vi "UHR-Fleezers Control (host) - 12.2.vi"() -> ()   [LabVIEW 2012] (continued)
            n266 = while {
              tunnel: w477 -> [w482]
              tunnel: w475 -> [w481]
              tunnel: w473 -> [w480]
              tunnel: w472 -> [w479]
              tunnel: w471 -> [w478]
              stop <- w483 stop-if-true
              n267 = event shown="[0] \"Pane\": Mouse Move" {
                selector: _ -> [_ _]
                dyn-events: _ -> [_ _]
                timeout: _ -> [_ _]
                tunnel: ["Force Manip Abort" w547] -> w483
                tunnel: w482 -> [w490 _]
                tunnel: w481 -> [w488 _]
                tunnel: w480 -> [w487 _]
                tunnel: w479 -> [w486 _]
                tunnel: w478 -> [w485 _]
                event Mouse Move {
                  n268 = event-data() -> ("Time"=w491:u32, "Coords"=w492:T7)  [unwired: 3 out]
                  n269 = Less?(x=w491, y=w490) -> (x < y?=w489:bool)
                  n270 = case "Makes sure old motion events prior to mouse click aren't used" shown="False" w489 {
                    tunnel: w492 -> [w534 _]
                    tunnel: w488 -> [w535 _]
                    tunnel: w487 -> [w512 _]
                    tunnel: w486 -> [w508 _]
                    tunnel: w485 -> [w507 _]
                    frame False {
                      n271 = Subtract(x=w534, y=w535) -> (x-y=w533:T7)
                      "Coords" <- w533
                      n272 = local read "Y RF Frequency Limits (MHz)"() -> (w493:T16)
                      n273 = To Double Precision Float(number=w533) -> (double precision float=w532:cluster{"Horizontal":dbl, "Vertical":dbl})
                      n274 = Multiply(x=cluster{"Horizontal":dbl, "Vertical":dbl} {"Horizontal"=-1.0, "Vertical"=1.0}, y="Manipulation Scaling") -> (x*y=w528:cluster{"Horizontal":dbl, "Vertical":dbl})
                      n275 = local read "X RF Frequency Limits (MHz)"() -> (w494:T16)
                      n276 = Multiply(x=w532, y=w528) -> (x*y=w530:cluster{"Horizontal":dbl, "Vertical":dbl})
                      n277 = Unbundle By Name(w530) -> ("Horizontal"=w525:dbl, "Vertical"=w529:dbl)
                      n278 = Unbundle By Name(w493) -> ("Maximum"=w496:dbl, "Minimum"=w495:dbl)
                      n279 = Boolean To (0,1)(Boolean="Manip. X?") -> (0, 1=w523:i16)
                      n280 = Boolean To (0,1)(Boolean="Manip. Y?") -> (0, 1=w520:i16)
                      n281 = local read "BD 1 Frequency 2 (MHz)"() -> (w510:dbl)
                      n282 = Multiply(x=w529, y=w520) -> (x*y=w522:dbl)
                      n283 = Multiply(x=w523, y=w525) -> (x*y=w526:dbl)
                      n284 = local read "BD 2 Frequency 2 (MHz)"() -> (w509:dbl)
                      n285 = Unbundle By Name(w494) -> ("Maximum"=w498:dbl, "Minimum"=w497:dbl)
                      n286 = Add(x=w507, y=w522) -> (x+y=w500:dbl)
                      n287 = Add(x=w508, y=w526) -> (x+y=w502:dbl)
                      n288 = In Range and Coerce(upper limit=w498, x=w502, lower limit=w497) -> (coerced(x)=w501:dbl)  [unwired: 1 out]
                      n289 = In Range and Coerce(upper limit=w496, x=w500, lower limit=w495) -> (coerced(x)=w499:dbl)  [unwired: 1 out]
                      n290 = Subtract(x=w501, y=w510) -> (x-y=w519:dbl)
                      n291 = Subtract(x=w499, y=w509) -> (x-y=w518:dbl)
                      n292 = Square(x=w519) -> (x^2=w517:dbl)
                      n293 = Square(x=w518) -> (x^2=w516:dbl)
                      n294 = Add(x=w517, y=w516) -> (x+y=w515:dbl)
                      n295 = Square Root(x=w515) -> (sqrt(x)=w511:dbl)
                      n296 = In Range and Coerce(upper limit="Limit Max (MHz)", x=w511, lower limit="Limit Min (MHz)") -> (In Range?=w504:bool)  [unwired: 1 out]
                      n297 = Not(x="Limits Enable") -> (.not. x?=w503:bool)
                      n298 = Or(x=w504, y=w503) -> (x .or. y?=w505:bool)
                      n299 = case shown="True" w505 {
                        tunnel: w512 -> [_ w545]
                        tunnel: w511 -> [_ w536]
                        tunnel: w501 -> [_ w543]
                        tunnel: w510 -> [_ w542]
                        tunnel: w499 -> [_ w541]
                        tunnel: w509 -> [_ w540]
                        tunnel: w494 -> [_ w538]
                        tunnel: w493 -> [_ w537]
                        frame False {
                        }
                        frame True {
                          n300 = local read "BD 1 Frequency 3 (MHz)"() -> (w544:dbl)
                          n301 = local read "BD 2 Frequency 3 (MHz)"() -> (w539:dbl)
                          n302 = local write "Trap Delta (MHz)"(w536) -> ()
                          n303 = call "set RF board frequency - interlace.vi"("Board 2 Frequency Limits"=w537, "Board 1 Frequency Limits"=w538, "FPGA VI Reference In"=w545, "Board 2 Frequency 3 (MHz)"=w539, "Board 1 Frequency 3 (MHz)"=w544, "Board 2 Frequency 2 (MHz)"=w540, "Board 2 Frequency 1 (MHz)"=w541, "Board 1 Frequency 2 (MHz)"=w542, "Board 1 Frequency 1  (MHz)"=w543) -> ()  [unwired: 1 in, 2 out]
                          n304 = local write "BD 2 Frequency 1 (MHz)"(w541) -> ()
                          n305 = local write "BD 1 Frequency 1 (MHz)"(w543) -> ()
                        }
                      }
                    }
                    frame True {
                    }
                  }
                }
                event Mouse Up {
                  n306 = event-data() -> ("Button"=w546:u16)  [unwired: 8 out]
                  n307 = case shown="3" w546 {
                    tunnel: [FALSE TRUE] -> w547
                    frame 0, Default {
                    }
                    frame 3 {
                      n308 = local read "Trap Delta (MHz)"() -> (w549:dbl)
                      n309 = property on="Initial delta (MHz)" class="DigNum (strict)"("Val(Sgnl)"=w549) -> ()  [unwired: 2 in, 2 out]
                      n310 = local write "Manipulating Trap"(FALSE ("Manipulating Trap")) -> ()
                    }
                  }
                }
              }
            }
          }
        }
      }
      event Mouse Move {
        n311 = event-data() -> ()  [unwired: 6 out]
      }
    }
    n312 = local read "Stop All"() -> (w365:bool)
    n313 = node-c288() -> ()  [unwired: 2 out]
  }
  n314 = node-c288() -> (w2:T21)  [unwired: 4 out]
  n315 = timed-loop "Run Scripts, including: stage motion" {
    tunnel: w129 -> [w558]
    tunnel: w128 -> [w559]
    tunnel: [w559] -> w127
    tunnel: [w558] -> w126
    timing: w124 -> [_]
    timing-out: [_] -> w123
    tunnel: w109 -> [w557]
    tunnel: w110 -> [w556]
    tunnel: w56 -> [w553]
    tunnel: w55 -> [w552]
    tunnel: w54 -> [w554]
    tunnel: w53 -> [w555]
    stop <- w560 stop-if-true
    n316 = node-c288() -> ()  [unwired: 1 in, 1 out]
    n317 = event shown="[1] \"Move to Position\": Value Change" {
      selector: _ -> [_ _ _ _ _ _ _ _ _ _ _ _ _ _ _ _ _ _ _]
      dyn-events: _ -> [_ _ _ _ _ _ _ _ _ _ _ _ _ _ _ _ _ _ _]
      timeout: _ -> [_ _ _ _ _ _ _ _ _ _ _ _ _ _ _ _ _ _ _]
      tunnel: ["Set Position" "Move to Position" _ _ "Read Harvard" _ _ _ _ _ _ "Got ADig bead" "Force FB Data\nScript" _ "Got DNA bead" "Take Stepping Data" _ "Take Detection Laser\nImage" _] -> _
      tunnel: [_ _ _ _ _ _ _ _ _ _ _ _ _ _ _ _ _ _ w1177] -> w560
      tunnel: w558 -> [w578 w586 w599 w629 _ w674 w714 w795 w824 w956 w982 _ w1018 _ _ _ _ _ _]
      tunnel: w559 -> [w579 w587 w600 w630 _ w675 w715 w796 w825 w957 w983 _ w1019 _ _ _ _ _ _]
      tunnel: w557 -> [_ _ _ _ w659 _ _ _ _ _ _ _ _ _ _ _ _ _ _]
      tunnel: w556 -> [_ _ _ _ w658 _ _ _ _ _ _ _ _ _ _ _ _ _ _]
      tunnel: w555 -> [_ _ _ _ _ _ _ _ _ _ _ _ _ _ _ _ _ _ _]
      tunnel: w554 -> [_ _ _ _ _ _ _ _ _ _ _ _ _ _ _ _ _ _ _]
      tunnel: w553 -> [_ _ _ _ _ _ _ _ _ _ _ _ _ _ _ _ _ _ _]
      tunnel: w552 -> [_ _ _ _ _ _ _ _ _ _ _ _ _ _ _ _ _ _ _]
      event "Set Position", "Set Position 2", "Set Position 3", "Set Position 4", "Set Position 5", "Set Position 1": Value Change {
        n318 = event-data() -> ()  [unwired: 1 in, 5 out]
        n319 = Build Array("Set Position 1", "Set Position 2", "Set Position 3", "Set Position 4", "Set Position 5") -> (w577:bool[])
        n320 = Boolean Array To Number(Boolean array=w577) -> (number=w576:u32)
        n321 = Logarithm Base 2(1:w576) -> (0:w568:dbl)
        n322 = call "Read Stage Position.vi"("error in"=w578, "VISA resource name in"=w579) -> ("Current Position"=w583:cluster{dbl, dbl, dbl}, "error out"=w582:errorcluster)  [unwired: 2 out]
        n323 = Decrement(x="Position") -> (x-1=w566:dbl)
        n324 = Greater Or Equal?(x=w568, y=0.0) -> (x >= y?=w569:bool)
        n325 = Cluster To Array(cluster=w583) -> (array=w580:dbl[])
        n326 = local write "Stage Control Serial Error"(w582) -> ()
        n327 = Select(t=w568, s=w569, f=w566) -> (s? t:f=w565:dbl)
        n328 = Increment(x=w565) -> (x+1=w564:dbl)
        n329 = Build Array (concatenate)(w564, w580) -> (w563:dbl[])
        n330 = Replace Array Subset(array="Saved Stage Positions", new element=w563, index (row)=w565) -> (w581:dbl[][])  [unwired: 1 in]
        n331 = local write "Saved Stage Positions"(w581) -> ()
      }
      event "Move to Position": Value Change {
        n332 = event-data() -> ()  [unwired: 1 in, 5 out]
        n333 = flat-sequence {
          tunnel: w587 -> [w591]
          tunnel: w586 -> [w590]
          frame #0 {
            n334 = local read "Saved Stage Positions"() -> (w593:dbl[][])
            n335 = local read "Position"() -> (w592:dbl)
            n336 = local write "Stage Moving"(TRUE ("Stage Moving")) -> ()
            n337 = call "move to saved stage position.vi"("error in"=w590, "Stage VISA resource name in"=w591, "Position"=w592, "Saved Stage Positions"=w593) -> ("error out"=w589:errorcluster)  [unwired: 1 out]
            n338 = local write "Stage Control Serial Error"(w589) -> ()
          }
          frame #1 {
            n339 = call <vilib>:"Beep.vi"() -> ()  [unwired: 3 in, 9 out]
            n340 = local write "Stage Moving"(FALSE ("Stage Moving")) -> ()
          }
        }
      }
      event "Move Cap. 1 (DNA Bottom)": Value Change {
        n341 = event-data() -> ()  [unwired: 1 in, 5 out]
        n342 = local write "Move Cap. 1 (DNA Bottom)"(FALSE ("Move Cap. 1 (DNA Right)")) -> ()
        n343 = flat-sequence {
          tunnel: w599 -> [w602]
          tunnel: w600 -> [w603]
          tunnel: [w603] -> w597
          tunnel: [w602] -> w596
          tunnel: w597 -> [w605]
          tunnel: w596 -> [w604]
          frame #0 {
            n344 = property on="Sample Channel\nFlow" class="Bool (strict)"("Val(Sgnl)"="Cap 1 Samp Flow ON") -> ()  [unwired: 2 in, 2 out]
          }
          frame #1 {
            n345 = local read "Saved Stage Positions"() -> (w615:dbl[][])
            n346 = local write "Stage Moving"(TRUE ("Stage Moving")) -> ()
            n347 = Array Subset(array=w615, index (row)=0 ("index"), length (row)=1 ("length"), index (col)=1 ("index"), length (col)=3 ("length")) -> (w612:dbl[][])
            n348 = Reshape Array(w612, 3 ("dimension size")) -> (w610:dbl[])
            n349 = Array To Cluster(array=w610) -> (cluster=w609:cluster{"[0]":dbl, "[1]":dbl, "[2]":dbl})
            n350 = call "Set Stage Position.vi"("Position"=w609, "error in"=w604, "VISA resource name in"=w605) -> ("error out"=w608:errorcluster)  [unwired: 2 out]
            n351 = local write "Stage Control Serial Error"(w608) -> ()
          }
          frame #2 {
            n352 = local write "Stage Moving"(FALSE ("Stage Moving")) -> ()
            n353 = case shown="True" "Cap 1 Flow ON" {
              frame False {
              }
              frame True {
                n354 = property on="Inject Pump 1" class="Bool (strict)"("Val(Sgnl)"=TRUE ("Value (Signaling)")) -> ()  [unwired: 2 in, 2 out]
              }
            }
            n355 = call <vilib>:"Beep.vi"() -> ()  [unwired: 3 in, 9 out]
          }
          frame #3 {
            n356 = property on="Sample Channel\nFlow" class="Bool (strict)"("Val(Sgnl)"=FALSE ("Value (Signaling)")) -> ()  [unwired: 2 in, 2 out]
            n357 = local read "Cap. 2 BD T1?\n(ADig T1, DNA T2)"() -> (w622:bool)
            n358 = case shown="True" w622 {
              tunnel: "Cap 1 T ON" -> [w624 w625]
              frame False {
                n359 = property on="Trap 1 (ON/OFF)" class="Bool (strict)"("Val(Sgnl)"=w624) -> ()  [unwired: 2 in, 2 out]
              }
              frame True {
                n360 = property on="Trap 2 (ON/OFF)" class="Bool (strict)"("Val(Sgnl)"=w625) -> ()  [unwired: 2 in, 2 out]
              }
            }
            n361 = property on="Got DNA bead" class="Bool"("Key Focus"=TRUE) -> ()  [unwired: 2 in, 2 out]
          }
        }
      }
      event "Move Cap. 2 (ADig Top)": Value Change {
        n362 = event-data() -> ()  [unwired: 1 in, 5 out]
        n363 = local write "Move Cap. 2 (ADig Top)"(FALSE ("Move Cap. 2 (ADig Left)")) -> ()
        n364 = flat-sequence {
          tunnel: w629 -> [w632]
          tunnel: w630 -> [w633]
          tunnel: [w633] -> w627
          tunnel: [w632] -> w626
          tunnel: w627 -> [w636]
          tunnel: w626 -> [w635]
          frame #0 {
            n365 = property on="Sample Channel\nFlow" class="Bool (strict)"("Val(Sgnl)"="Cap 2 Samp Flow ON") -> ()  [unwired: 2 in, 2 out]
          }
          frame #1 {
            w634 = FALSE ("Value (Signaling)")
            n366 = local read "Saved Stage Positions"() -> (w646:dbl[][])
            n367 = local write "Stage Moving"(TRUE ("Stage Moving")) -> ()
            n368 = Array Subset(array=w646, index (row)=1 ("index"), length (row)=1 ("length"), index (col)=1 ("index"), length (col)=3 ("length")) -> (w643:dbl[][])
            n369 = Reshape Array(w643, 3 ("dimension size")) -> (w641:dbl[])
            n370 = property on="Trap 1 (ON/OFF)" class="Bool (strict)"("Val(Sgnl)"=w634) -> ()  [unwired: 2 in, 2 out]
            n371 = property on="Trap 1 (ON/OFF)" class="Bool (strict)"("Val(Sgnl)"=w634) -> ()  [unwired: 2 in, 2 out]
            n372 = Array To Cluster(array=w641) -> (cluster=w640:cluster{"[0]":dbl, "[1]":dbl, "[2]":dbl})
            n373 = call "Set Stage Position.vi"("Position"=w640, "error in"=w635, "VISA resource name in"=w636) -> ("error out"=w639:errorcluster)  [unwired: 2 out]
            n374 = local write "Stage Control Serial Error"(w639) -> ()
          }
          frame #2 {
            n375 = local write "Stage Moving"(FALSE ("Stage Moving")) -> ()
            n376 = call <vilib>:"Beep.vi"() -> ()  [unwired: 3 in, 9 out]
            n377 = case shown="True" "Cap 2 Flow ON" {
              frame False {
              }
              frame True {
                n378 = property on="Inject Pump 3" class="Bool (strict)"("Val(Sgnl)"=TRUE ("Value (Signaling)")) -> ()  [unwired: 2 in, 2 out]
              }
            }
          }
          frame #3 {
            n379 = property on="Sample Channel\nFlow" class="Bool (strict)"("Val(Sgnl)"=FALSE ("Value (Signaling)")) -> ()  [unwired: 2 in, 2 out]
            n380 = case shown="False" "Cap. 2 BD T1?\n(ADig T1, DNA T2)" {
              tunnel: "Cap 2 T ON" -> [w655 w656]
              frame False {
                n381 = property on="Trap 2 (ON/OFF)" class="Bool (strict)"("Val(Sgnl)"=w655) -> ()  [unwired: 2 in, 2 out]
              }
              frame True {
                n382 = property on="Trap 1 (ON/OFF)" class="Bool (strict)"("Val(Sgnl)"=w656) -> ()  [unwired: 2 in, 2 out]
              }
            }
            n383 = property on="Got ADig bead" class="Bool"("Key Focus"=TRUE) -> ()  [unwired: 2 in, 2 out]
          }
        }
      }
      event "Read Harvard": Value Change {
        n384 = event-data() -> ()  [unwired: 1 in, 5 out]
        n385 = Concatenate Strings("write buffer", "\r") -> (w661:string)
        n386 = VISA Write(VISA resource name=w659, write buffer=w661, error in (no error)=w658) -> (VISA resource name out=w670:refnum<visa-resource-name>, error out=w669:errorcluster)  [unwired: 1 out]
        n387 = stacked-sequence {
          tunnel: [w673] -> w668
          tunnel: w670 -> [w673]
          tunnel: w669 -> [w672]
          tunnel: [w672] -> w663
          frame #0 {
            n388 = Wait (ms)(milliseconds to wait=50) -> ()  [unwired: 1 out]
          }
        }
        n389 = property class="Instr"(reference=w668, error in=w663) -> (reference out=w667:refnum<visa-resource-name>, error out=w665:errorcluster, "Serial Settings:Number of Bytes at Serial Port"=w666:u32)
        "Serial Settings:Number of Bytes at Serial Port" <- w666
        n390 = VISA Read(VISA resource name=w667, byte count=w666, error in (no error)=w665) -> (read buffer=w664:string)  [unwired: 3 out]
        "read buffer" <- w664
        n391 = Fract/Exp String To Number(string=w664) -> ()  [unwired: 5 out]
      }
      event "+z", "-z": Value Change {
        n392 = event-data() -> ()  [unwired: 1 in, 5 out]
        n393 = flat-sequence {
          tunnel: w674 -> [w696]
          tunnel: w675 -> [w676]
          frame #0 {
            n394 = call "Read Stage Position.vi"("error in"=w696, "VISA resource name in"=w676) -> ("Current Position"=w681:cluster{dbl, dbl, dbl}, "error out"=w694:errorcluster, "VISA resource name out"=w695:refnum<visa-resource-name>)  [unwired: 1 out]
            n395 = local read "Saved Stage Positions"() -> (w705:dbl[][])
            n396 = Divide(x="z nudge increment (um)", y=1000.0) -> (x/y=w693:dbl)
            n397 = Boolean To (0,1)(Boolean="+z") -> (0, 1=w685:i16)
            n398 = Boolean To (0,1)(Boolean="-z") -> (0, 1=w686:i16)
            n399 = Array Subset(array=w705, index (row)=1 ("index"), length (row)=1 ("length"), index (col)=1 ("index"), length (col)=3 ("length")) -> (w702:dbl[][])
            n400 = Multiply(x=w685, y=w693) -> (x*y=w689:dbl)
            n401 = Multiply(x=w686, y=w693) -> (x*y=w687:dbl)
            n402 = Unbundle(w681) -> (w679:dbl, w678:dbl, w682:dbl)
            n403 = Negate(x=w687) -> (-x=w688:dbl)
            n404 = Reshape Array(w702, 3 ("dimension size")) -> (w700:dbl[])
            n405 = Add(x=w689, y=w688) -> (x+y=w690:dbl)
            n406 = Array To Cluster(array=w700) -> ()  [unwired: 1 out]
            n407 = Add(x=w690, y=w682) -> (x+y=w680:dbl)
            n408 = Bundle(cluster=w681, w679, w678, w680) -> (w677:cluster{dbl, dbl, dbl})
            n409 = call "Set Stage Position.vi"("Position"=w677, "error in"=w694, "VISA resource name in"=w695) -> ("error out"=w699:errorcluster)  [unwired: 2 out]
            n410 = local write "Stage Moving"(TRUE ("Stage Moving")) -> ()
            n411 = local write "Stage Control Serial Error"(w699) -> ()
          }
          frame #1 {
            n412 = local write "Stage Moving"(FALSE ("Stage Moving")) -> ()
            n413 = call <vilib>:"Beep.vi"() -> ()  [unwired: 3 in, 9 out]
          }
        }
      }
      event "Cal/Data Acq. Spot": Value Change {
        n414 = event-data() -> ()  [unwired: 1 in, 5 out]
        n415 = flat-sequence {
          tunnel: w714 -> [w718]
          tunnel: w715 -> [w719]
          tunnel: [w719] -> w711
          tunnel: [w718] -> w710
          tunnel: w711 -> [w724]
          tunnel: w710 -> [w723]
          tunnel: ["Cal @ (MHz)"] -> w708
          tunnel: [w728] -> w712
          tunnel: w708 -> [w728]
          tunnel: w712 -> [w737]
          tunnel: ["W/ Offset 1"] -> w709
          tunnel: w712 -> [w758]
          tunnel: w709 -> [w756]
          frame #0 {
            n416 = property on="Sample Channel\nFlow" class="Bool (strict)"("Val(Sgnl)"="Daq spot flow on") -> ()  [unwired: 2 in, 2 out]
            n417 = Wait (ms)(milliseconds to wait=u32 250) -> ()  [unwired: 1 out]
          }
          frame #1 {
            n418 = local read "Saved Stage Positions"() -> (w721:dbl[][])
            n419 = property on="Trap Delta (MHz)" class="DigNum (strict)"("Val(Sgnl)"="Cal @ (MHz)") -> ()  [unwired: 2 in, 2 out]
            n420 = local write "Stage Moving"(TRUE ("Stage Moving")) -> ()
            n421 = call "move to saved stage position.vi"("error in"=w723, "Stage VISA resource name in"=w724, "Position"="Cal Stage Position", "Saved Stage Positions"=w721) -> ("error out"=w722:errorcluster)  [unwired: 1 out]
            n422 = local write "Stage Control Serial Error"(w722) -> ()
          }
          frame #2 {
            n423 = local write "Stage Moving"(FALSE ("Stage Moving")) -> ()
            n424 = property on="Sample Channel\nFlow" class="Bool (strict)"("Val(Sgnl)"="Flow ON during cal?") -> ()  [unwired: 2 in, 2 out]
            n425 = call <vilib>:"Beep.vi"() -> ()  [unwired: 3 in, 9 out]
          }
          frame #3 {
            n426 = Wait (ms)(milliseconds to wait=u32 1000) -> ()  [unwired: 1 out]
          }
          frame #4 {
            n427 = property on="Save Calibration" class="Bool (strict)"("Val(Sgnl)"=TRUE ("Value (Signaling)")) -> ()  [unwired: 2 in, 2 out]
          }
          frame #5 {
            n428 = Wait (ms)(milliseconds to wait=u32 2000) -> ()  [unwired: 1 out]
          }
          frame #6 {
            # "Check to see if \nsaving done"
            n429 = while {
              stop <- w733 stop-if-true
              n430 = local read "Saving..."() -> (w734:bool)
              n431 = Wait (ms)(milliseconds to wait=u32 100) -> ()  [unwired: 1 out]
              n432 = Not(x=w734) -> (.not. x?=w733:bool)
            }
          }
          frame #7 {
            n433 = case shown="True" "W/ Offset 1" {
              tunnel: w737 -> [_ w738]
              frame False {
              }
              frame True {
                n434 = stacked-sequence {
                  tunnel: w738 -> [_ _ _ _ _ _ _ w755]
                  frame #0 {
                    n435 = property on="Trap Delta (MHz)" class="DigNum (strict)"("Val(Sgnl)"="Offset 1 Start (MHz)") -> ()  [unwired: 2 in, 2 out]
                    n436 = Replace Array Subset(array=u32[] [0] ("Index Values"), new element="Offset 1 Set", index=0) -> (w739:u32[])
                    n437 = property on="Saved AOD Raster Scan Parameter Sets" class="Arr (strict)"("Index Values"=w739) -> ()  [unwired: 2 in, 2 out]
                  }
                  frame #1 {
                    n438 = Wait (ms)(milliseconds to wait=u32 200) -> ()  [unwired: 1 out]
                  }
                  frame #2 {
                    n439 = property on="Load parameters" class="Bool (strict)"("Val(Sgnl)"=TRUE ("Value (Signaling)")) -> ()  [unwired: 2 in, 2 out]
                  }
                  frame #3 {
                    n440 = Wait (ms)(milliseconds to wait=u32 200) -> ()  [unwired: 1 out]
                  }
                  frame #4 {
                    n441 = property on="Trap Raster Scan" class="Bool (strict)"("Val(Sgnl)"=TRUE ("Value (Signaling)")) -> ()  [unwired: 2 in, 2 out]
                  }
                  frame #5 {
                    n442 = Wait (ms)(milliseconds to wait=u32 2000) -> ()  [unwired: 1 out]
                  }
                  frame #6 {
                    n443 = while {
                      stop <- w752 stop-if-true
                      n444 = local read "Raster Scanning..."() -> (w754:bool)
                      n445 = local read "Saving..."() -> (w750:bool)
                      n446 = Wait (ms)(milliseconds to wait=u32 100) -> ()  [unwired: 1 out]
                      n447 = Not(x=w750) -> (.not. x?=w749:bool)
                      n448 = Not(x=w754) -> (.not. x?=w751:bool)
                      n449 = And(x=w751, y=w749) -> (x .and. y?=w752:bool)
                    }
                  }
                  frame #7 {
                    n450 = property on="Trap Delta (MHz)" class="DigNum (strict)"("Val(Sgnl)"=w755) -> ()  [unwired: 2 in, 2 out]
                  }
                }
              }
            }
          }
          frame #8 {
            n451 = local read "Save ave N"() -> (w757:dbl)
            n452 = case shown="False" "W/ Offset 2" {
              tunnel: w758 -> [_ w765]
              tunnel: w757 -> [_ w764]
              tunnel: w756 -> [w760 _]
              frame False {
                n453 = case shown="False" w760 {
                  frame False {
                    n454 = Multiply(x="Cal read wait (s)", y=u32 1000 ("milliseconds to wait")) -> (x*y=w762:u32)
                    n455 = Wait (ms)(milliseconds to wait=w762) -> ()  [unwired: 1 out]
                  }
                  frame True {
                  }
                }
              }
              frame True {
                n456 = stacked-sequence {
                  tunnel: w765 -> [_ _ _ _ _ _ _ _ _ w786 _ _]
                  tunnel: w764 -> [_ _ _ _ _ _ _ _ _ w784 _ _]
                  frame #0 {
                    n457 = property on="Save ave N" class="DigNum (strict)"("Val(Sgnl)"=1.0 ("Value (Signaling)")) -> ()  [unwired: 2 in, 2 out]
                  }
                  frame #1 {
                    n458 = Wait (ms)(milliseconds to wait=u32 500) -> ()  [unwired: 1 out]
                  }
                  frame #2 {
                    n459 = property on="Trap Delta (MHz)" class="DigNum (strict)"("Val(Sgnl)"="Offset 2 Start (MHz)") -> ()  [unwired: 2 in, 2 out]
                    n460 = Replace Array Subset(array=u32[] [0] ("Index Values"), new element="Offset 2 Set", index=0) -> (w770:u32[])
                    n461 = property on="Saved AOD Raster Scan Parameter Sets" class="Arr (strict)"("Index Values"=w770) -> ()  [unwired: 2 in, 2 out]
                  }
                  frame #3 {
                    n462 = Wait (ms)(milliseconds to wait=u32 500) -> ()  [unwired: 1 out]
                  }
                  frame #4 {
                    n463 = property on="Load parameters" class="Bool (strict)"("Val(Sgnl)"=TRUE ("Value (Signaling)")) -> ()  [unwired: 2 in, 2 out]
                  }
                  frame #5 {
                    n464 = Wait (ms)(milliseconds to wait=u32 500) -> ()  [unwired: 1 out]
                  }
                  frame #6 {
                    n465 = property on="Trap Raster Scan" class="Bool (strict)"("Val(Sgnl)"=TRUE ("Value (Signaling)")) -> ()  [unwired: 2 in, 2 out]
                  }
                  frame #7 {
                    n466 = Wait (ms)(milliseconds to wait=u32 2000) -> ()  [unwired: 1 out]
                  }
                  frame #8 {
                    n467 = while {
                      stop <- w779 stop-if-true
                      n468 = local read "Raster Scanning..."() -> (w782:bool)
                      n469 = local read "Saving..."() -> (w780:bool)
                      n470 = Wait (ms)(milliseconds to wait=u32 100) -> ()  [unwired: 1 out]
                      n471 = Not(x=w780) -> (.not. x?=w778:bool)
                      n472 = Not(x=w782) -> (.not. x?=w781:bool)
                      n473 = And(x=w781, y=w778) -> (x .and. y?=w779:bool)
                    }
                  }
                  frame #9 {
                    n474 = property on="Trap Delta (MHz)" class="DigNum (strict)"("Val(Sgnl)"=w786) -> ()  [unwired: 2 in, 2 out]
                    n475 = property on="Saved AOD Raster Scan Parameter Sets" class="Arr (strict)"("Index Values"=u32[] [0]) -> ()  [unwired: 2 in, 2 out]
                    n476 = property on="Save ave N" class="DigNum (strict)"("Val(Sgnl)"=w784) -> ()  [unwired: 2 in, 2 out]
                  }
                  frame #10 {
                    n477 = Wait (ms)(milliseconds to wait=u32 500) -> ()  [unwired: 1 out]
                  }
                  frame #11 {
                    n478 = property on="Load parameters" class="Bool (strict)"("Val(Sgnl)"=TRUE ("Value (Signaling)")) -> ()  [unwired: 2 in, 2 out]
                  }
                }
              }
            }
          }
          frame #9 {
            n479 = property on="Read Cal" class="Bool (strict)"("Val(Sgnl)"=TRUE ("Value (Signaling)")) -> ()  [unwired: 2 in, 2 out]
          }
          frame #10 {
            n480 = Wait (ms)(milliseconds to wait=u32 1000) -> ()  [unwired: 1 out]
          }
          frame #11 {
            n481 = property on="Fish for Tether" class="Bool (strict)"("Val(Sgnl)"=TRUE ("Value (Signaling)")) -> ()  [unwired: 2 in, 2 out]
          }
        }
        n482 = local write "Cal/Data Acq. Spot"(FALSE ("Cal/Data Acq. Spot")) -> ()
      }
      event "Dump Beads": Value Change {
        n483 = event-data() -> ()  [unwired: 1 in, 5 out]
        n484 = flat-sequence {
          tunnel: ["Dump spot flow on?"] -> w792
          tunnel: [w803] -> w793
          tunnel: w792 -> [w803]
          tunnel: w796 -> [w808]
          tunnel: w795 -> [w807]
          tunnel: [w805] -> w794
          tunnel: w793 -> [w805]
          tunnel: w794 -> [w818]
          frame #0 {
            w797 = FALSE ("Value (Signaling)")
            n485 = local read "Saving..."() -> (w799:bool)
            n486 = local write "Dump Beads"(FALSE ("Dump Beads")) -> ()
            n487 = property on="Inject Pump 3" class="Bool (strict)"("Val(Sgnl)"=w797) -> ()  [unwired: 2 in, 2 out]
            n488 = property on="Inject Pump 1" class="Bool (strict)"("Val(Sgnl)"=w797) -> ()  [unwired: 2 in, 2 out]
            n489 = local write "Stop Saving"(w799) -> ()
          }
          frame #1 {
            w800 = FALSE ("Fl. Triggered...")
            n490 = case shown="True" "Dump spot flow on?" {
              frame False {
              }
              frame True {
                n491 = property on="Sample Channel\nFlow" class="Bool (strict)"("Val(Sgnl)"=TRUE ("Stage Moving")) -> ()  [unwired: 2 in, 2 out]
              }
            }
            n492 = local write "Fl. Triggered..."(w800) -> ()
            n493 = local write "Tether"(w800) -> ()
            n494 = property on="Green Laser ON/Interlacing" class="Bool (strict)"("Val(Sgnl)"=w800) -> ()  [unwired: 2 in, 2 out]
            n495 = property on="Trap Pos. FB ON" class="Bool (strict)"("Val(Sgnl)"=w800) -> ()  [unwired: 2 in, 2 out]
            n496 = property on="Trap Trig. Fl." class="Bool (strict)"("Val(Sgnl)"=w800) -> ()  [unwired: 2 in, 2 out]
            n497 = property on="Fl. Triggered..." class="Bool (strict)"("Val(Sgnl)"=w800) -> ()  [unwired: 2 in, 2 out]
            n498 = property on="Dip for Protein" class="Bool (strict)"("Val(Sgnl)"=w800) -> ()  [unwired: 2 in, 2 out]
            n499 = property on="Pause dwell" class="Bool (strict)"("Val(Sgnl)"=w800) -> ()  [unwired: 2 in, 2 out]
          }
          frame #2 {
            n500 = property on="Trap Pos. FB Offset Factor" class="DigNum (strict)"("Val(Sgnl)"=i64 0 ("Value (Signaling)")) -> ()  [unwired: 2 in, 2 out]
          }
          frame #3 {
            n501 = local read "Saved Stage Positions"() -> (w809:dbl[][])
            n502 = local write "Stage Moving"(TRUE ("Stage Moving")) -> ()
            n503 = Array Subset(array=w809, index (row)=3 ("index"), length (row)=1 ("length"), index (col)=1 ("index"), length (col)=3 ("length")) -> (w814:dbl[][])
            n504 = Reshape Array(w814, 3 ("dimension size")) -> (w812:dbl[])
            n505 = Array To Cluster(array=w812) -> (cluster=w811:cluster{"[0]":dbl, "[1]":dbl, "[2]":dbl})
            n506 = call "Set Stage Position.vi"("Position"=w811, "error in"=w807, "VISA resource name in"=w808) -> ()  [unwired: 3 out]
          }
          frame #4 {
            w819 = FALSE ("Value (Signaling)")
            n507 = case shown="True" w818 {
              frame False {
              }
              frame True {
                n508 = property on="Sample Channel\nFlow" class="Bool (strict)"("Val(Sgnl)"=FALSE ("Stage Moving")) -> ()  [unwired: 2 in, 2 out]
              }
            }
            n509 = property on="Trap 1 (ON/OFF)" class="Bool (strict)"("Val(Sgnl)"=w819) -> ()  [unwired: 2 in, 2 out]
            n510 = property on="Trap 2 (ON/OFF)" class="Bool (strict)"("Val(Sgnl)"=w819) -> ()  [unwired: 2 in, 2 out]
            n511 = call <vilib>:"Beep.vi"() -> ()  [unwired: 3 in, 9 out]
          }
          frame #5 {
            n512 = property on="Move Cap. 2 (ADig Top)" class="Bool (strict)"("Val(Sgnl)"=TRUE ("Value (Signaling)")) -> ()  [unwired: 2 in, 2 out]
            n513 = property on="Tab Control" class="TabCtl (strict)"("Val(Sgnl)"=T4."Status" ("Value (Signaling)")) -> ()  [unwired: 2 in, 2 out]
          }
        }
      }
      event "Dip for Protein": Value Change {
        n514 = event-data() -> ()  [unwired: 1 in, 5 out]
        n515 = case shown="True" "Dip for Protein" {
          tunnel: w825 -> [_ w827]
          tunnel: w824 -> [_ w826]
          frame False {
          }
          frame True {
            n516 = while {
              tunnel: w827 -> [w838]
              tunnel: w826 -> [w837]
              i -> [w832]
              stop <- w834 stop-if-true
              n517 = Increment(x=w832) -> (x+1=→"Dip #":i32)
              n518 = flat-sequence {
                tunnel: w837 -> [w849]
                tunnel: w838 -> [w850]
                tunnel: [w850] -> w842
                tunnel: [w849] -> w841
                tunnel: [w843] -> w828
                tunnel: [w855] -> w836
                tunnel: [w856] -> w835
                tunnel: w842 -> [w857]
                tunnel: w841 -> [w858]
                tunnel: [w853] -> w829
                tunnel: w828 -> [w853]
                tunnel: [w866] -> w840
                tunnel: w836 -> [w866]
                tunnel: [w865] -> w839
                tunnel: w835 -> [w865]
                tunnel: [w862] -> w833
                tunnel: [w861] -> w830
                tunnel: w829 -> [w861]
                tunnel: w839 -> [w886]
                tunnel: w840 -> [w887]
                tunnel: w833 -> [w888]
                tunnel: w830 -> [w885]
                tunnel: [w944] -> w834
                frame #0 {
                  n519 = local read "Trap Pos. FB ON"() -> (w843:bool)
                  n520 = Compound Arithmetic op=AND("Flow ON\nduring dip?", "FB OFF when \nflow ON", w843) -> (w844:bool)
                  n521 = case shown="True" "Move trap \nbefore dip move?" {
                    frame False {
                    }
                    frame True {
                      n522 = property on="Trap Delta (MHz)" class="DigNum (strict)"("Val(Sgnl)"="Dipping Delta (MHz)") -> ()  [unwired: 2 in, 2 out]
                    }
                  }
                  n523 = property on="Green Laser ON/Interlacing" class="Bool (strict)"("Val(Sgnl)"="Green ON\nbefore dip?") -> ()  [unwired: 2 in, 2 out]
                  n524 = property on="Sample Channel\nFlow" class="Bool (strict)"("Val(Sgnl)"="Flow ON\nduring dip?") -> ()  [unwired: 2 in, 2 out]
                  n525 = case shown="True" w844 {
                    frame False {
                    }
                    frame True {
                      n526 = property on="Trap Pos. FB ON" class="Bool (strict)"("Val(Sgnl)"=FALSE ("Value (Signaling)")) -> ()  [unwired: 2 in, 2 out]
                    }
                  }
                }
                frame #1 {
                  n527 = local read "Saved Stage Positions"() -> (w860:dbl[][])
                  n528 = local write "Cancel dwell"(FALSE ("Cancel dwell")) -> ()
                  n529 = call "move to saved stage position.vi"("error in"=w858, "Stage VISA resource name in"=w857, "Position"="Dip Stage \nPosition", "Saved Stage Positions"=w860) -> ("VISA resource name out"=w855:refnum<visa-resource-name>, "error out"=w856:errorcluster)
                }
                frame #2 {
                  n530 = node-c288() -> (w864:T21)  [unwired: 4 in]
                  n531 = timed-loop {
                    timing: w864 -> [_]
                    timing-out: [_] -> w863
                    tunnel: [w870] -> w862
                    i -> [w867]
                    stop <- w871 stop-if-true
                    n532 = node-c288() -> ()  [unwired: 1 in, 1 out]
                    n533 = Greater Or Equal?(x=w867, y="Dip Duration (s)") -> (x >= y?=w879:bool)
                    n534 = local read "Dip for Protein"() -> (w872:bool)
                    n535 = local read "Dump Beads"() -> (w869:bool)
                    n536 = local read "Cancel dwell"() -> (w878:bool)
                    n537 = local read "Pause dwell"() -> (w875:bool)
                    n538 = Not(x=w872) -> (.not. x?=w877:bool)
                    n539 = Compound Arithmetic op=OR(w878, w879, w877) -> (w876:bool)
                    n540 = Select(t=FALSE, s=w875, f=w876) -> (s? t:f=w873:bool)
                    n541 = Not(x=w869) -> (.not. x?=w868:bool)
                    n542 = node-c288() -> ()  [unwired: 1 in, 1 out]
                    n543 = And(x=w872, y=w868) -> (x .and. y?=w870:bool)
                    n544 = Or(x=w873, y=w869) -> (x .or. y?=w871:bool)
                    "Dip Time (s)" <- w867
                  }
                  n545 = node-c288(w863) -> ()  [unwired: 1 out]
                }
                frame #3 {
                  n546 = case shown="True" w888 {
                    tunnel: w887 -> [_ w893]
                    tunnel: w886 -> [_ w892]
                    tunnel: w885 -> [_ w889]
                    frame False {
                    }
                    frame True {
                      n547 = flat-sequence {
                        tunnel: w892 -> [w897]
                        tunnel: w893 -> [w898]
                        tunnel: [w898] -> w891
                        tunnel: [w897] -> w890
                        tunnel: w889 -> [w894]
                        tunnel: w891 -> [w908]
                        tunnel: w890 -> [w907]
                        tunnel: w889 -> [w916]
                        frame #0 {
                          n548 = local read "Sample Channel\nFlow"() -> (w896:bool)
                          n549 = case shown="True" w896 {
                            tunnel: "Flow ON \nduring return\nfrom dip?" -> [w899 w902]
                            tunnel: w894 -> [_ w901]
                            frame False {
                              n550 = case shown="True" w899 {
                                frame False {
                                }
                                frame True {
                                n551 = property on="Sample Channel\nFlow" class="Bool (strict)"("Val(Sgnl)"=TRUE ("Value (Signaling)")) -> ()  [unwired: 2 in, 2 out]
                                }
                              }
                            }
                            frame True {
                              n552 = case shown="False" w902 {
                                tunnel: w901 -> [w903 _]
                                frame False {
                                n553 = property on="Trap Pos. FB ON" class="Bool (strict)"("Val(Sgnl)"=w903) -> ()  [unwired: 2 in, 2 out]
                                n554 = property on="Sample Channel\nFlow" class="Bool (strict)"("Val(Sgnl)"=FALSE ("Value (Signaling)")) -> ()  [unwired: 2 in, 2 out]
                                }
                                frame True {
                                }
                              }
                            }
                          }
                        }
                        frame #1 {
                          # "For turning on green laser before stage reaches lower spot"
                          n555 = case shown="True" "Green ON\nafter start\nreturn?" {
                            frame False {
                            }
                            frame True {
                              n556 = flat-sequence {
                                frame #0 {
                                n557 = Multiply(x="Green delay after \nstart return (s)", y=1000.0) -> (x*y=w913:dbl)
                                n558 = Wait (ms)(milliseconds to wait=w913) -> ()  [unwired: 1 out]
                                }
                                frame #1 {
                                n559 = property on="Green Laser ON/Interlacing" class="Bool (strict)"("Val(Sgnl)"=TRUE ("Value (Signaling)")) -> ()  [unwired: 2 in, 2 out]
                                }
                              }
                            }
                          }
                          n560 = local read "Saved Stage Positions"() -> (w911:dbl[][])
                          n561 = local write "Cancel dwell"(FALSE ("Cancel dwell")) -> ()
                          n562 = call "move to saved stage position.vi"("error in"=w907, "Stage VISA resource name in"=w908, "Position"="Return Stage \nPosition", "Saved Stage Positions"=w911) -> ("error out"=w909:errorcluster)  [unwired: 1 out]
                          n563 = local write "Stage Control Serial Error"(w909) -> ()
                        }
                        frame #2 {
                          n564 = property on="Trap Pos. FB ON" class="Bool (strict)"("Val(Sgnl)"=w916) -> ()  [unwired: 2 in, 2 out]
                          n565 = case shown="True" "Green ON \nafter return?" {
                            frame False {
                            }
                            frame True {
                              n566 = property on="Green Laser ON/Interlacing" class="Bool (strict)"("Val(Sgnl)"=TRUE ("Value (Signaling)")) -> ()  [unwired: 2 in, 2 out]
                            }
                          }
                          n567 = case shown="True" "Move trap after return?" {
                            frame False {
                            }
                            frame True {
                              n568 = property on="Trap Delta (MHz)" class="DigNum (strict)"("Val(Sgnl)"="Dip Trap Delta 2 (MHz)") -> ()  [unwired: 2 in, 2 out]
                            }
                          }
                          n569 = case shown="True" "Save data after return?" {
                            frame False {
                            }
                            frame True {
                              n570 = property on="Start Saving" class="Bool (strict)"("Val(Sgnl)"=TRUE ("Value (Signaling)")) -> ()  [unwired: 2 in, 2 out]
                            }
                          }
                          n571 = property on="Sample Channel\nFlow" class="Bool (strict)"("Val(Sgnl)"="Flow ON\nduring daq?") -> ()  [unwired: 2 in, 2 out]
                        }
                        frame #3 {
                          n572 = node-c288() -> (w925:T21)  [unwired: 4 in]
                          n573 = timed-loop {
                            timing: w925 -> [_]
                            timing-out: [_] -> w924
                            i -> [w926]
                            stop <- w928 stop-if-true
                            n574 = node-c288() -> ()  [unwired: 1 in, 1 out]
                            n575 = local read "Dump Beads"() -> (w927:bool)
                            n576 = Greater Or Equal?(x=w926, y="Dwell Duration (s)") -> (x >= y?=w933:bool)
                            n577 = local read "Dip for Protein"() -> (w930:bool)
                            n578 = Not(x=w930) -> (.not. x?=w929:bool)
                            n579 = Compound Arithmetic op=OR(w933, "Cancel dwell", w929) -> (w932:bool)
                            n580 = node-c288() -> ()  [unwired: 1 in, 1 out]
                            n581 = Select(t=FALSE, s="Pause dwell", f=w932) -> (s? t:f=w935:bool)
                            n582 = Or(x=w935, y=w927) -> (x .or. y?=w928:bool)
                            "Dwell Time (s)" <- w926
                          }
                          n583 = node-c288(w924) -> ()  [unwired: 1 out]
                        }
                      }
                    }
                  }
                }
                frame #4 {
                  n584 = local read "Dip for Protein"() -> (w945:bool)
                  n585 = local read "Dump Beads"() -> (w942:bool)
                  n586 = local write "Cancel dwell"(FALSE ("Cancel dwell")) -> ()
                  n587 = Not(x=w945) -> (.not. x?=w946:bool)
                  n588 = Not(x="Cont. Repeat Dipping?") -> (.not. x?=w948:bool)
                  n589 = Compound Arithmetic op=OR(w946, w948, w942) -> (w944:bool)
                }
              }
            }
          }
        }
      }
      event "Profile": Value Change {
        n590 = event-data() -> ()  [unwired: 1 in, 5 out]
        n591 = flat-sequence {
          tunnel: w957 -> [w960]
          tunnel: w956 -> [w968]
          tunnel: [w962] -> w955
          tunnel: [w961] -> w954
          tunnel: [w959] -> w952
          tunnel: [w958] -> w949
          tunnel: w955 -> [w975]
          tunnel: w954 -> [w974]
          tunnel: [w972] -> w953
          tunnel: w952 -> [w973]
          tunnel: [w971] -> w951
          tunnel: [w970] -> w950
          tunnel: w949 -> [w970]
          tunnel: w953 -> [w979]
          tunnel: w951 -> [w978]
          tunnel: w950 -> [w977]
          frame #0 {
            n592 = call "Read Stage Position.vi"("error in"=w968, "VISA resource name in"=w960) -> ("Current Position"=w958:cluster{dbl, dbl, dbl}, "error out"=w961:errorcluster, "VISA resource name out"=w959:refnum<visa-resource-name>)  [unwired: 1 out]
            "Current Position" <- w958
            n593 = local write "Stage Control Serial Error"(w961) -> ()
            n594 = Unbundle(w958) -> (w965:dbl, w967:dbl, w963:dbl)
            n595 = Add(x=w967, y="Y change (mm)") -> (x+y=w964:dbl)
            n596 = Bundle(w965, w964, w963) -> (w962:cluster{dbl, dbl, dbl})  [unwired: 1 in]
          }
          frame #1 {
            # "move to new position and start saving"
            n597 = local write "Stage Moving"(TRUE ("Stage Moving")) -> ()
            n598 = local write "Start Saving"(TRUE ("Start Saving")) -> ()
            n599 = call "Set Stage Position.vi"("Position"=w975, "error in"=w974, "VISA resource name in"=w973) -> ("error out"=w971:errorcluster, "VISA resource name out"=w972:refnum<visa-resource-name>)  [unwired: 1 out]
          }
          frame #2 {
            # "go back to start"
            n600 = call "Set Stage Position.vi"("Position"=w977, "error in"=w978, "VISA resource name in"=w979) -> ()  [unwired: 3 out]
          }
          frame #3 {
            # "stop saving"
            n601 = local write "Stop Saving"(TRUE ("Stop Saving")) -> ()
            n602 = local write "Stage Moving"(FALSE ("Stage Moving")) -> ()
          }
        }
      }
      event "Move to Position 1", "Move to Position 2", "Move to Position 3", "Move to Position 4", "Move to Position 5", "Lower Ch. Cap.": Value Change {
        n603 = event-data() -> ()  [unwired: 1 in, 5 out]
        n604 = Or(x="Move to Position 5", y="Lower Ch. Cap.") -> (x .or. y?=w985:bool)
        n605 = Build Array("Move to Position 1", "Move to Position 2", "Move to Position 3", "Move to Position 4", w985) -> (w988:bool[])
        n606 = Boolean Array To Number(Boolean array=w988) -> (number=w987:u32)
        n607 = Logarithm Base 2(1:w987) -> (0:w986:dbl)
        n608 = flat-sequence {
          tunnel: w986 -> [w997]
          tunnel: w983 -> [w995]
          tunnel: w982 -> [w994]
          frame #0 {
            n609 = local read "Saved Stage Positions"() -> (w1005:dbl[][])
            n610 = Array Subset(array=w1005, index (row)=w997, length (row)=1 ("length"), index (col)=1 ("index"), length (col)=3 ("length")) -> (w1002:dbl[][])
            n611 = Reshape Array(w1002, 3 ("dimension size")) -> (w1000:dbl[])
            n612 = Array To Cluster(array=w1000) -> (cluster=w999:cluster{"[0]":dbl, "[1]":dbl, "[2]":dbl})
            n613 = call "Set Stage Position.vi"("Position"=w999, "error in"=w994, "VISA resource name in"=w995) -> ("error out"=w998:errorcluster)  [unwired: 2 out]
            n614 = local write "Stage Moving"(TRUE ("Stage Moving")) -> ()
            n615 = local write "Stage Control Serial Error"(w998) -> ()
          }
          frame #1 {
            n616 = local write "Stage Moving"(FALSE ("Stage Moving")) -> ()
            n617 = call <vilib>:"Beep.vi"() -> ()  [unwired: 3 in, 9 out]
          }
        }
      }
      event "Got ADig bead": Value Change {
        n618 = event-data() -> ()  [unwired: 1 in, 5 out]
        n619 = flat-sequence {
          frame #0 {
            n620 = local read "Cap 1 Samp Flow ON"() -> (w1009:bool)
            n621 = case shown="True" w1009 {
              frame False {
              }
              frame True {
                n622 = property on="Sample Channel\nFlow" class="Bool (strict)"("Val(Sgnl)"=TRUE ("Value (Signaling)")) -> ()  [unwired: 2 in, 2 out]
              }
            }
          }
          frame #1 {
            n623 = property on="Inject Pump 3" class="Bool (strict)"("Val(Sgnl)"=FALSE ("Value (Signaling)")) -> ()  [unwired: 2 in, 2 out]
          }
          frame #2 {
            n624 = property on="Move Cap. 1 (DNA Bottom)" class="Bool (strict)"("Val(Sgnl)"=TRUE ("Value (Signaling)")) -> ()  [unwired: 2 in, 2 out]
          }
        }
      }
      event "Force FB Data\nScript": Value Change {
        n625 = event-data() -> ()  [unwired: 1 in, 5 out]
        n626 = flat-sequence {
          tunnel: w1018 -> [w1022]
          tunnel: w1019 -> [w1023]
          tunnel: [w1023] -> w1014
          tunnel: [w1022] -> w1013
          tunnel: w1014 -> [w1026]
          tunnel: w1013 -> [w1025]
          tunnel: ["Trap Trig Fl."] -> w1015
          tunnel: [w1051] -> w1016
          tunnel: w1015 -> [w1051]
          tunnel: [w1055] -> w1017
          tunnel: w1016 -> [w1055]
          tunnel: w1017 -> [w1057]
          frame #0 {
            n627 = property on="Trap Delta (MHz)" class="DigNum (strict)"("Val(Sgnl)"="Trap Delta Before Moving") -> ()  [unwired: 2 in, 2 out]
          }
          frame #1 {
            n628 = local read "Saved Stage Positions"() -> (w1028:dbl[][])
            n629 = local write "FB Trap Pos Offset"(0.0 ("FB Trap Pos Offset")) -> ()
            n630 = property on="Trap Pos. FB Offset Factor" class="DigNum (strict)"("Val(Sgnl)"=i64 0 ("Value (Signaling)")) -> ()  [unwired: 2 in, 2 out]
            n631 = local write "Stage Moving"(TRUE ("Stage Moving")) -> ()
            n632 = call "move to saved stage position.vi"("error in"=w1025, "Stage VISA resource name in"=w1026, "Position"="Stage Position To Establish FB", "Saved Stage Positions"=w1028) -> ("error out"=w1024:errorcluster)  [unwired: 1 out]
            n633 = local write "Stage Control Serial Error"(w1024) -> ()
          }
          frame #2 {
            n634 = call <vilib>:"Beep.vi"() -> ()  [unwired: 3 in, 9 out]
            n635 = Multiply(x="Wait (s)", y=u32 1000 ("milliseconds to wait")) -> (x*y=w1035:u32)
            n636 = property on="Trap Delta (MHz)" class="DigNum (strict)"("Val(Sgnl)"="Starting \nTrap Delta (MHz)") -> ()  [unwired: 2 in, 2 out]
            n637 = local write "Stage Moving"(FALSE ("Stage Moving")) -> ()
            n638 = Wait (ms)(milliseconds to wait=w1035) -> ()  [unwired: 1 out]
            n639 = property on="Tab Control 2" class="TabCtl (strict)"("Val(Sgnl)"=T6."Feedback on Trap Position" ("Value (Signaling)")) -> ()  [unwired: 2 in, 2 out]
            n640 = property on="Tab Control" class="TabCtl (strict)"("Val(Sgnl)"=T4."Trap Control (RF)" ("Value (Signaling)")) -> ()  [unwired: 2 in, 2 out]
          }
          frame #3 {
            n641 = property on="Set Reading to\nSetpoint" class="Bool (strict)"("Val(Sgnl)"=TRUE ("Value (Signaling)")) -> ()  [unwired: 2 in, 2 out]
            n642 = Wait (ms)(milliseconds to wait=u32 500) -> ()  [unwired: 1 out]
          }
          frame #4 {
            n643 = property on="Trap Pos. FB ON" class="Bool (strict)"("Val(Sgnl)"=TRUE ("Value (Signaling)")) -> ()  [unwired: 2 in, 2 out]
            n644 = Wait (ms)(milliseconds to wait=u32 250) -> ()  [unwired: 1 out]
          }
          frame #5 {
            n645 = case shown="False" "Trap Trig Fl." {
              frame False {
                n646 = case shown="True" "Green ON after FB ON?" {
                  selector: "Green ON after FB ON?" -> [_ w1050]
                  frame False {
                  }
                  frame True {
                    n647 = property on="Green Laser ON/Interlacing" class="Bool (strict)"("Val(Sgnl)"=w1050) -> ()  [unwired: 2 in, 2 out]
                  }
                }
              }
              frame True {
              }
            }
            n648 = case shown="True" "Remove Action Offset" {
              tunnel: TRUE ("Value (Signaling)") -> [w1047 w1048]
              frame False {
                n649 = property on="Remove Unwinding Offset" class="Bool (strict)"("Val(Sgnl)"=w1047) -> ()  [unwired: 2 in, 2 out]
              }
              frame True {
                n650 = property on="Remove Action Offset" class="Bool (strict)"("Val(Sgnl)"=w1048) -> ()  [unwired: 2 in, 2 out]
              }
            }
